vi "Client TLS Config Control.vi"() -> ()   [LabVIEW 2020]
uses:
  TCP Comms/Cert Chain.ctl
  TCP Comms/TinyTCP.lvlib
  TCP Comms/Client TLS Config.ctl
panel:
  in  "Client TLS Config":T1
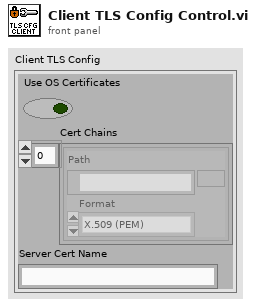
[diagram p1: front panel]
types:
  T1 = typedef "TinyTCP.lvlib/Client TLS Config.ctl" = cluster{"Use OS Certificates":bool, "Cert Chains":T2[], "Server Cert Name":string}
  T2 = typedef "TinyTCP.lvlib/Cert Chain.ctl" = cluster{"Path":path, "Format":enum32{"X.509 (PEM)"}}
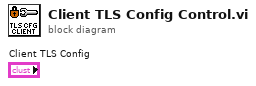
[diagram p0: block diagram]
diagram:
